vi "read_write.vi"(4 "offx":dbl, 5 "offy":dbl, 6 "driftvar":dbl, 7 "Write Result":bool, 8 "ypos":dbl, 9 "xpos":dbl, 10 "reference in":refnum<vi>, 11 "Path in":refnum<vi>) -> ()   [LabVIEW 2019]
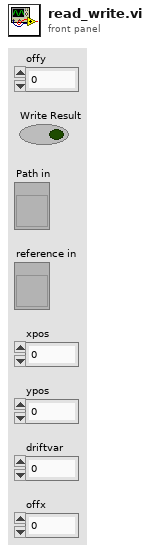
[diagram p1: front panel]
types:
  T1 = enum16{"open", "replace", "create", "open or create", "replace or create", "replace or create with confirmation"}
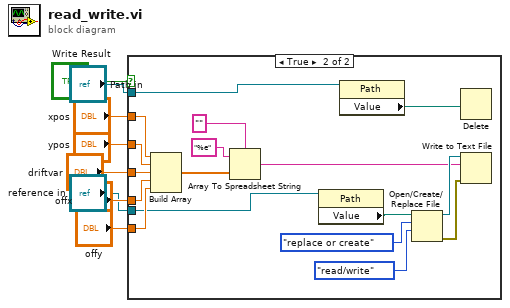
[diagram p0: block diagram]
diagram:
  n1 = case shown="True" "Write Result" {
    tunnel: "xpos" -> [_ w18]
    tunnel: "ypos" -> [_ w17]
    tunnel: "driftvar" -> [_ w15]
    tunnel: "offx" -> [_ w14]
    tunnel: "offy" -> [_ w13]
    tunnel: "Path in" -> [_ w10]
    tunnel: "reference in" -> [_ w9]
    frame False {
    }
    frame True {
      n2 = Build Array(w18, w17, w15, w14, w13) -> (w21:dbl[])
      n3 = Array To Spreadsheet String(delimiter (Tab)="", array=w21, 3:"%e" ("format string")) -> (spreadsheet string=w20:string)
      n4 = property class="Path"(reference=w9) -> ("Value"=w11:path)  [unwired: 1 in, 2 out]
      n5 = property class="Path"(reference=w10) -> ("Value"=w12:path)  [unwired: 1 in, 2 out]
      n6 = Open/Create/Replace File(file path (use dialog)=w11, operation (0:open)=T1."replace or create", access (0:read/write)=enum16{"read/write", "read-only", "write-only"}."read/write") -> (refnum out=w23:refnum<file>, error out=w22:errorcluster)  [unwired: 3 in, 1 out]
      n7 = Delete(path (use dialog)=w12) -> ()  [unwired: 4 in, 3 out]
      n8 = Write to Text File(file (use dialog)=w23, text=w20, error in=w22) -> ()  [unwired: 1 in, 3 out]
    }
  }
